vi "getVariableHeaderLength.vi"(11 "ControlPacket in":refnum<class "ControlPacket.lvclass">) -> (1 "size definitive":bool, 2 "VariableHeader size":u32, 3 "ControlPacket out":refnum<class "ControlPacket.lvclass">)   [LabVIEW 2013, in "MQTT_Control_Packets.lvlib" / "ControlPacket.lvclass"]
uses:
  ControlPacket.lvclass
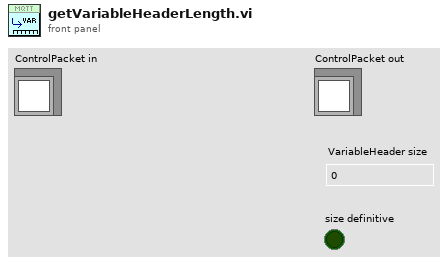
[diagram p1: front panel]
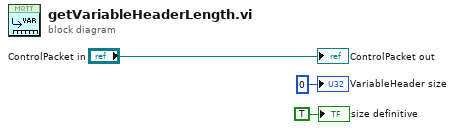
[diagram p0: block diagram]
diagram:
  "ControlPacket out" <- "ControlPacket in"
  "VariableHeader size" <- u32 0 ("VariableHeader size")
  "size definitive" <- TRUE ("size definitive")
